vi "Initialize.vi"(8 "error in":errorcluster) -> (0 "error out":errorcluster, 3 "SECS Data Class out":refnum<class "SECS Data Class.lvclass">)   [LabVIEW 2020, in "SECS Communication.lvlib" / "SECS Data Class.lvclass"]
uses:
  SECS Data Class.lvclass
  SECS Data Class.lvclass/SECS Data Class.ctl
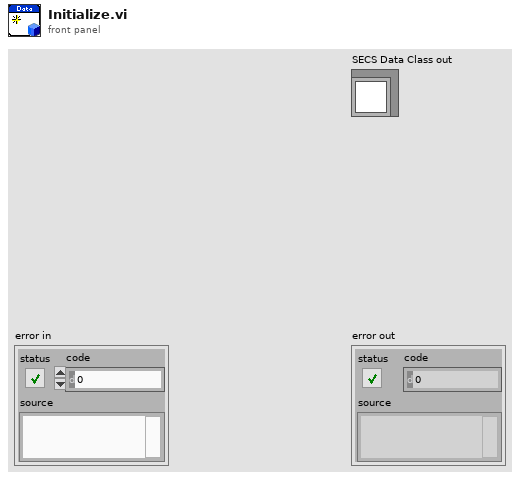
[diagram p1: front panel]
types:
  T1 = typedef "SECS Communication.lvlib/SECS Data Class.lvclass/SVID Data.ctl" = cluster{"SVID":u32, "Name":string, "Description":string, "Format Code":T2, "Unit":string, "Source":string, "Data":variant}
  T2 = typedef "SECS Communication.lvlib/SECS-II Class.lvclass/Format Code.ctl" = enum16{"L", "A", "B", "Boolean", "J", "I1", "I2", "I4", "I8", "U1", "U2", "U4", "U8", "F4", "F8", "Char"}
  T3 = typedef "SECS Communication.lvlib/SECS Data Class.lvclass/ECID Data.ctl" = cluster{"ECID":u32, "Name":string, "Description":string, "Format Code":T2, "Unit":string, "Max":dbl, "Min":dbl, "Default":string, "Source":string, "Data":variant}
  T4 = typedef "SECS Communication.lvlib/SECS Data Class.lvclass/ALID Data.ctl" = cluster{"Enable":bool, "ALID":u32, "Name":string, "Description":string, "Source":string, "Status":enum16{"Null", "Normal", "Abnormal", "Warning"}}
  T5 = typedef "SECS Communication.lvlib/SECS Data Class.lvclass/CEID Data.ctl" = cluster{"Enable":bool, "CEID":u32, "Name":string, "Description":string, "RPTID":u32[], "Dynamic":bool}
  T6 = typedef "SECS Communication.lvlib/SECS Data Class.lvclass/RPTID Data.ctl" = cluster{"RPTID":u32, "Report Information":string[], "Dynamic":bool}
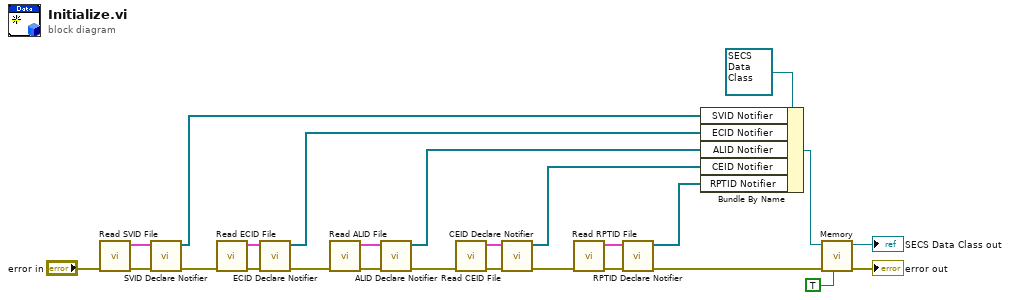
[diagram p0: block diagram]
diagram:
  n1 = call "Read SVID File.vi"("error in"="error in") -> ("error out"=w26:errorcluster, "SVID Data"=w25:T1[])  [unwired: 9 in]
  n2 = call "SVID Declare Notifier.vi"("error in"=w26, "SVID Data"=w25) -> ("error out"=w19:errorcluster, "SVID Notifier"=w16:refnum<notifier>[])  [unwired: 8 in]
  n3 = call "Read ECID File.vi"("error in"=w19) -> ("error out"=w24:errorcluster, "ECID Data"=w23:T3[])  [unwired: 9 in]
  n4 = call "ECID Declare Notifier.vi"("error in"=w24, "ECID Data"=w23) -> ("error out"=w18:errorcluster, "ECID Notifier"=w15:refnum<notifier>[])  [unwired: 8 in]
  n5 = call "Read ALID File.vi"("error in"=w18) -> ("error out"=w20:errorcluster, "ALID Data"=w21:T4[])  [unwired: 9 in]
  n6 = call "ALID Declare Notifier.vi"("error in"=w20, "ALID Data"=w21) -> ("error out"=w13:errorcluster, "ALID Notifier"=w14:refnum<notifier>[])  [unwired: 8 in]
  n7 = call "Read CEID File.vi"("error in"=w13) -> ("error out"=w12:errorcluster, "CEID Data"=w11:T5[])  [unwired: 9 in]
  n8 = call "CEID Declare Notifier.vi"("error in"=w12, "CEID Data"=w11) -> ("error out"=w3:errorcluster, "CEID Notifier"=w10:refnum<notifier>[])  [unwired: 8 in]
  n9 = call "Read RPTID File.vi"("error in"=w3) -> ("error out"=w4:errorcluster, "RPTID Data"=w5:T6[])  [unwired: 9 in]
  n10 = call "RPTID Declare Notifier.vi"("error in"=w4, "RPTID Data"=w5) -> ("error out"=w1:errorcluster, "RPTID Notifier"=w2:refnum<notifier>[])  [unwired: 8 in]
  n11 = Bundle By Name(cluster=refnum<class "SECS Data Class.lvclass"> refnum ("SECS Data Class in"), "SVID Notifier"=w16, "ECID Notifier"=w15, "ALID Notifier"=w14, "CEID Notifier"=w10, "RPTID Notifier"=w2) -> (w9:refnum<class "SECS Data Class.lvclass">)
  n12 = call "Memory.vi"("Put"=TRUE, "error in (no error)"=w1, "SECS Data Class in"=w9) -> ("error out"=→"error out":errorcluster, "SECS Data Class out"=→"SECS Data Class out":refnum<class "SECS Data Class.lvclass">)  [unwired: 7 in]
